vi "Galvo_Init.vi"(6 "Sample Mode":i32(ring)=10123 items=["Finite Samples"=10178, "Continuous Samples"=10123, "Hardware Timed Single Point"=12522], 7 "samples per channel":i32=1000, 8 "error in":errorcluster, 10 "Signal array":dynamicdata[](array[waveform]), 11 "Galvo_Input":T1={"Sample Rate"=1000.0, "Sample Clock Source"="OnboardClock", "Max Voltage"=5.0, "Min Voltage"=-5.0, "Physical Channel(s)"="Dev1/ao0"}) -> (0 "error out":errorcluster, 2 "Actual Sample Rate":dbl=1000.0 format="%0.2f", 3 "task out":refnum<k21>)   [LabVIEW 2014]
doc: "This SubVI is used to initiate a galvo mirror."
uses:
  TypeDef/GalvoInput.ctl
  <vilib>/DAQmx/write.llb/DAQmx Write (Analog 1D Wfm NChan NSamp).vi
  <vilib>/DAQmx/create/channels.llb/DAQmx Create Channel (AO-Voltage-Basic).vi
  <vilib>/DAQmx/configure/timing.llb/DAQmx Timing (Sample Clock).vi
  <vilib>/DAQmx/miscellaneous.llb/DAQmx Fill In Error Info.vi
  <resource>/objmgr/daqmx.rc
panel:
  # "This SubVI is used to initiate a galvo mirror."
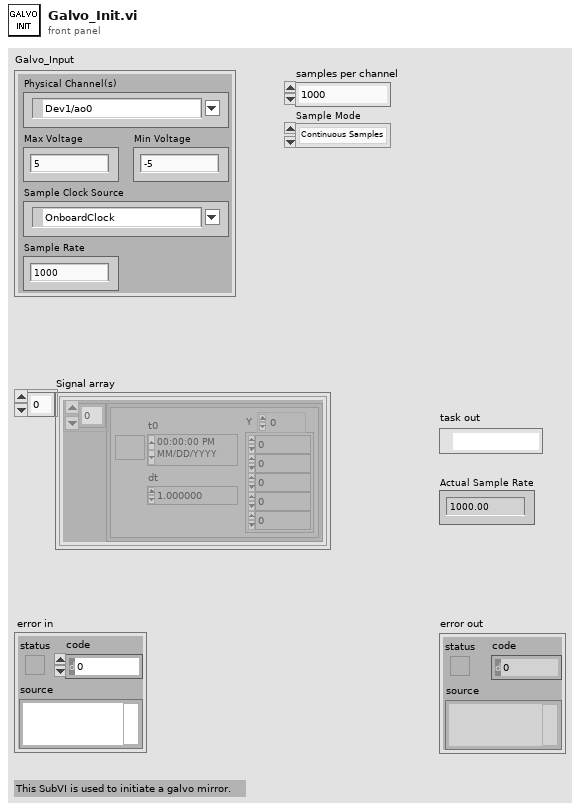
[diagram p1: front panel]
types:
  T1 = typedef "GalvoInput.ctl" = cluster{"Sample Rate":dbl, "Sample Clock Source":tag, "Max Voltage":dbl, "Min Voltage":dbl, "Physical Channel(s)":tag}
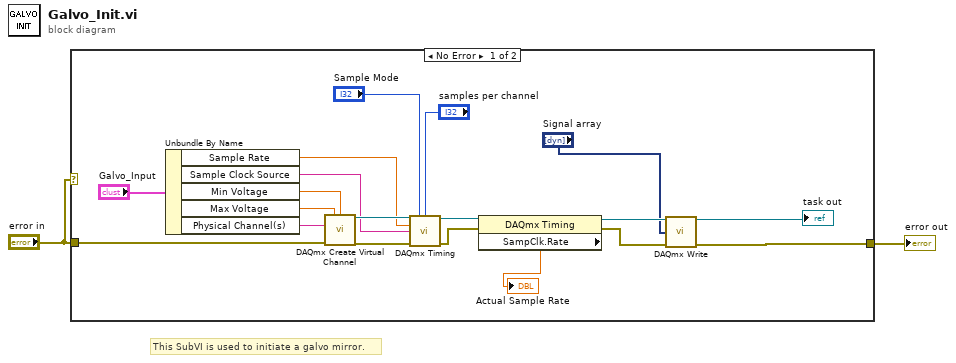
[diagram p0: block diagram]
diagram:
  # "This SubVI is used to initiate a galvo mirror."
  n1 = case shown="No Error" "error in" {
    tunnel: [w5 w22] -> w2
    tunnel: "error in" -> [w13 w22]
    frame No Error {
      n2 = Unbundle By Name("Galvo_Input") -> ("Sample Rate"=w11:dbl, "Sample Clock Source"=w10:tag, "Min Voltage"=w9:dbl, "Max Voltage"=w8:dbl, "Physical Channel(s)"=w7:tag)
      n3 = call-poly <vilib>:"DAQmx Create Virtual Channel.vi"("maximum value"=w8, "minimum value"=w9, "physical channels"=w7, "error in"=w13) -> ("task out"=w18:refnum<k21>, "error out"=w17:errorcluster)  [unwired: 10 in]
      n4 = call-poly <vilib>:"DAQmx Timing.vi"("task/channels in"=w18, "sample mode"="Sample Mode", "samples per channel"="samples per channel", "rate"=w11, "source"=w10, "error in"=w17) -> ("task out"=w14:refnum<k21>, "error out"=w15:errorcluster)  [unwired: 8 in]
      n5 = property class="DAQmx Timing"(reference=w14, error in=w15) -> (reference out=w20:refnum<k21>, error out=w21:errorcluster, "SampClk.Rate"=→"Actual Sample Rate":dbl)
      n6 = call-poly <vilib>:"DAQmx Write.vi"("task/channels in"=w20, "data"="Signal array", "error in"=w21) -> ("task out"=→"task out":refnum<k21>, "error out"=w5:errorcluster)  [unwired: 10 in, 1 out]
    }
    frame Error {
    }
  }
  "error out" <- w2
